vi "UI Destroy.vi"(8 "error in (no error)":errorcluster, 11 "Button_UI in":refnum<class "Button_UI.lvclass">) -> (0 "error out":errorcluster, 3 "Button_UI out":refnum<class "Button_UI.lvclass">)   [LabVIEW 2015, in "Button_UI.lvclass"]
uses:
  Button_UI.lvclass
  GUI Control/GUI Control.lvclass
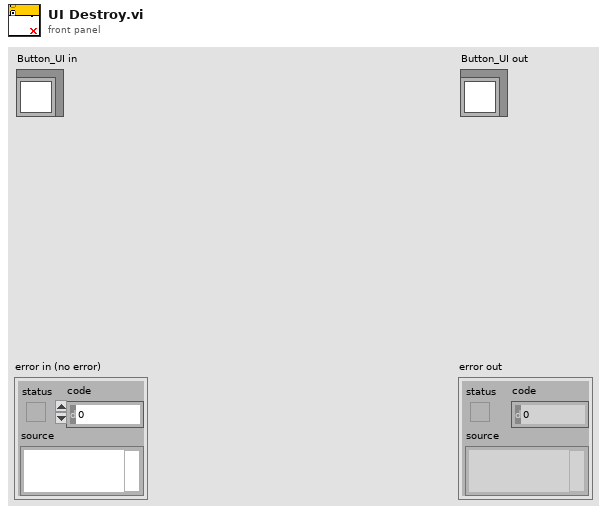
[diagram p1: front panel]
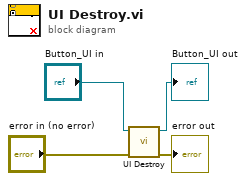
[diagram p0: block diagram]
diagram:
  n1 = call-parent "UI Destroy.vi"("error in (no error)"="error in (no error)", "GUI Control in"="Button_UI in") -> ("error out"=→"error out":errorcluster, "GUI Control out"=→"Button_UI out":refnum<class "Button_UI.lvclass">)  [unwired: 8 in]
